vi "onGetPlatanoVarietal.vi"(8 "error in (no error)":errorcluster, 11 "Platano.CarayaTestSuite in":refnum<class "Platano.CarayaTestSuite.lvclass">) -> (0 "error out":errorcluster, 2 "Varietal":string, 3 "Platano.CarayaTestSuite out":refnum<class "Platano.CarayaTestSuite.lvclass">)   [LabVIEW 2021, in "Banana.Caraya.lvlib" / "Platano.CarayaTestSuite.lvclass"]
uses:
  Platano.CarayaTestSuite.lvclass
  Platano.CarayaTestSuite.lvclass/Platano.CarayaTestSuite.ctl
  Bananas/Platano/Platano.lvclass
  Leaf.Properties.Suite/Leaf.Properties.Suite.lvclass
  Bananas/Leaf/Leaf.lvclass
  C:/Repositories/LVOS/Bananas/lv-src/Banana.Caraya/Leaf.Properties/Leaf.Properties.lvclass
  C:/Program Files (x86)/National Instruments/LabVIEW 2021/vi.lib/addons/_JKI Toolkits/Caraya/classes/Properties/Properties.lvclass
  C:/Repositories/LVOS/Bananas/lv-src/Bananas/Leaf/Leaf.lvclass
  C:/Repositories/LVOS/Bananas/lv-src/Bananas/Leaf.TestSuite/Leaf.TestSuite.lvclass
  C:/Repositories/LVOS/Bananas/lv-src/Banana.Caraya/Leaf.Properties.Suite/Leaf.Properties.Suite.lvclass
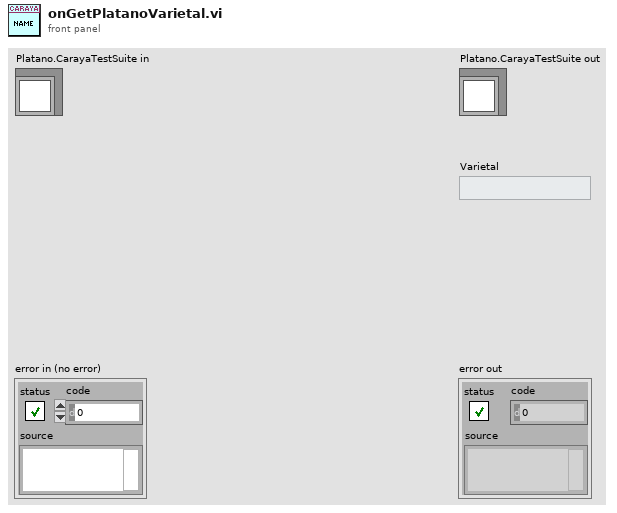
[diagram p1: front panel]
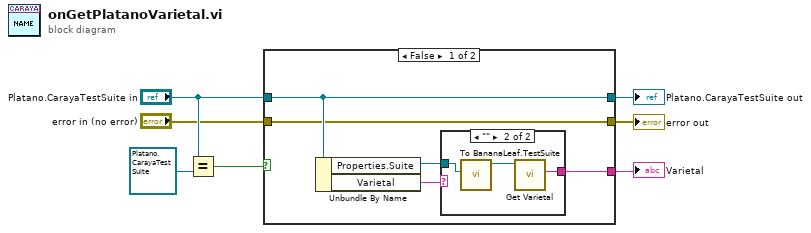
[diagram p0: block diagram]
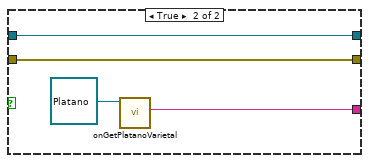
[diagram p3: hidden frame]
diagram:
  n1 = Equal?(x="Platano.CarayaTestSuite in", y=refnum<class "Platano.CarayaTestSuite.lvclass"> refnum) -> (x = y?=w4:bool)
  n2 = case shown="False" w4 {
    tunnel: [w9 w19] -> w7
    tunnel: "Platano.CarayaTestSuite in" -> [w12 w17]
    tunnel: [w12 w17] -> w3
    tunnel: "error in (no error)" -> [w11 w18]
    tunnel: [w11 w18] -> w1
    frame False {
      n3 = Unbundle By Name(w12) -> ("Properties.Suite"=w10:refnum<class "Properties.Suite.lvclass">, "Varietal"=w8:string)
      n4 = case shown="\"\"" w8 {
        selector: w8 -> [w13 _]
        tunnel: w10 -> [_ w16]
        tunnel: [w13 w14] -> w9
        frame Default {
        }
        frame "" {
          n5 = call "To BananaLeaf.TestSuite.vi"("Properties.Suite"=w16) -> ("Leaf.Properties.TestSuite out"=w15:refnum<class "Leaf.Properties.Suite.lvclass">)  [unwired: 10 in]
          n6 = call "Get Varietal.vi"("Leaf in"=w15) -> ("Varietal"=w14:string)  [unwired: 8 in, 2 out]
        }
      }
    }
    frame True {
      n7 = call-dynamic "onGetPlatanoVarietal.vi"("Platano in"=refnum<class "Platano.lvclass"> refnum ("Bananas.lvlib:Platano.lvclass")) -> ("Varietal"=w19:string)  [unwired: 8 in, 2 out]
    }
  }
  "error out" <- w1
  "Platano.CarayaTestSuite out" <- w3
  "Varietal" <- w7
